vi "getFrequency.vi"(0 "FrequencyCounter in":refnum<class "FrequencyCounter.lvclass">, 1 "error in (no error)":errorcluster) -> (2 "FrequencyCounter out":refnum<class "FrequencyCounter.lvclass">, 3 "Frequency":string, 4 "error out":errorcluster)   [LabVIEW 2009, in "Hardware.lvlib" / "frequencyCounters.lvlib" / "FrequencyCounter.lvclass"]
uses:
  FrequencyCounter.lvclass
  FrequencyCounter.lvclass/FrequencyCounter.ctl
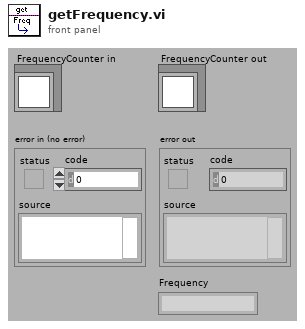
[diagram p1: front panel]
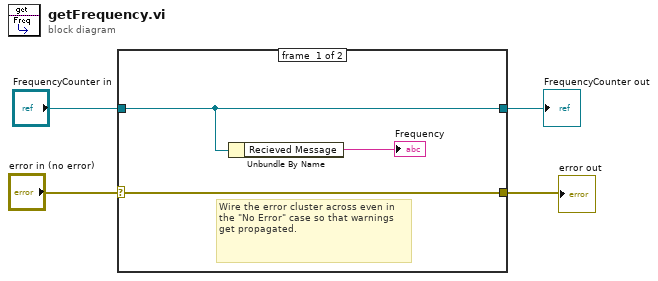
[diagram p0: block diagram]
diagram:
  n1 = case shown="No Error" "error in (no error)" {
    selector: "error in (no error)" -> [w7 w8]
    tunnel: [w7 w8] -> w3
    tunnel: [w6 w9] -> w1
    tunnel: "FrequencyCounter in" -> [w6 w9]
    frame #0 {
      # "Wire the error cluster across even in the \"No Error\" case so that warnings get propagated."
      n2 = Unbundle By Name(w6) -> ("Recieved Message"=→"Frequency":string)
    }
    frame #1 {
    }
  }
  "error out" <- w3
  "FrequencyCounter out" <- w1
